vi "New Buffer with data.vi"(7 "#bytes per timestamp":i32, 9 "New Buffer Size (#timestamps)":i32, 10 "Values (buffered, rotated)":u8[](array[numeric]), 11 "Timestamps (buffered, rotated)":u64[](array[numeric])) -> (0 "Full?":bool, 1 "index":i32, 2 "Values (new buffer)":u8[](array[numeric]), 3 "Timestamps (new buffer)":u64[](array[numeric]))   [LabVIEW 2021, in "Ring Buffer Time Series Data.lvlib"]
uses:
  Ring Buffer Time Series Data.lvlib
  Enforce array size multiple timestamps.vi
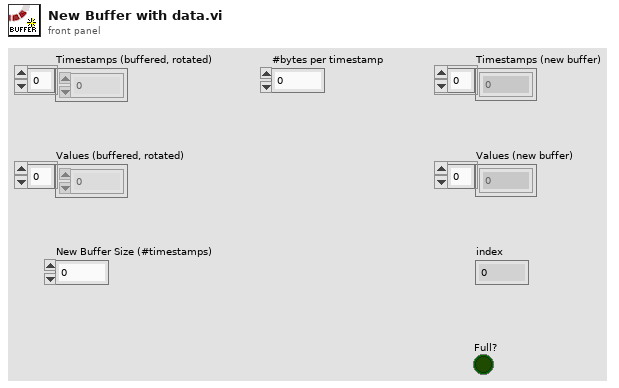
[diagram p1: front panel]
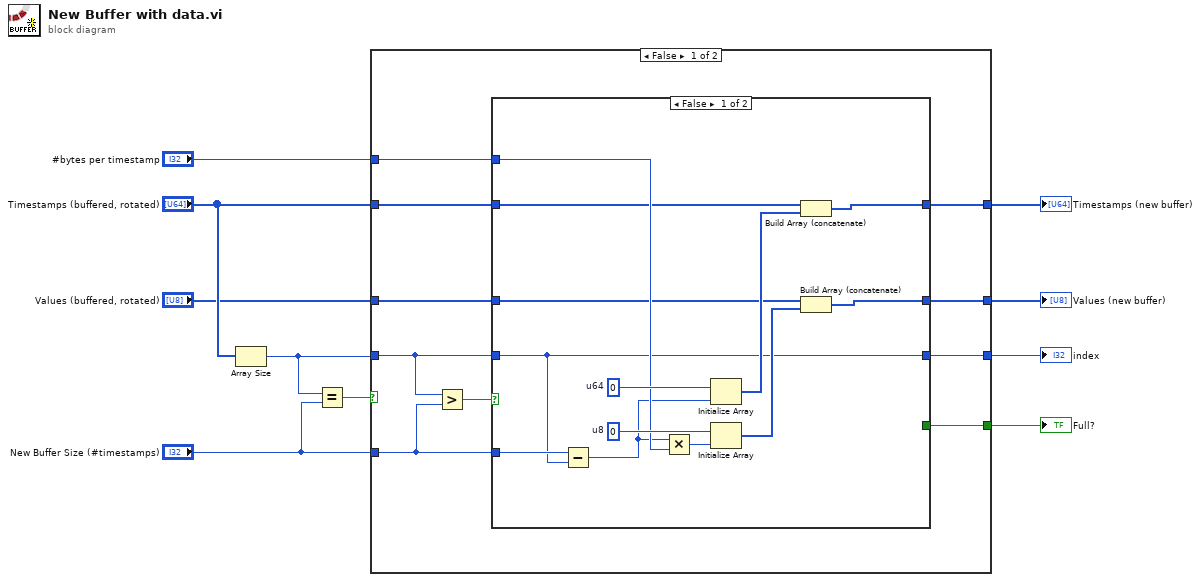
[diagram p0: block diagram]
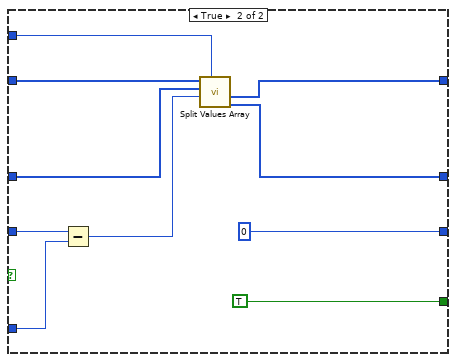
[diagram p2: hidden frame]
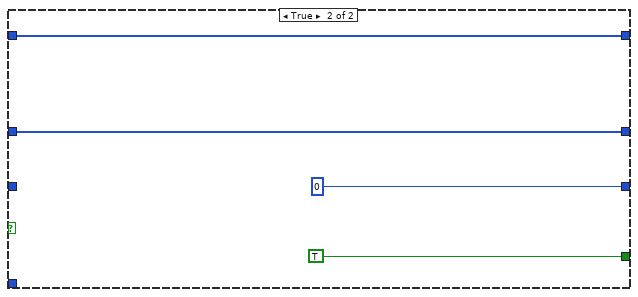
[diagram p3: hidden frame]
diagram:
  n1 = Array Size(array="Timestamps (buffered, rotated)") -> (size(s)=w4:i32)
  n2 = Equal?(x=w4, y="New Buffer Size (#timestamps)") -> (x = y?=w10:bool)
  n3 = case shown="False" w10 {
    tunnel: "Timestamps (buffered, rotated)" -> [w19 w47]
    tunnel: [w18 w47] -> w8
    tunnel: "Values (buffered, rotated)" -> [w16 w46]
    tunnel: [w15 w46] -> w6
    tunnel: [w12 TRUE ("Full?")] -> w5
    tunnel: w4 -> [w11 _]
    tunnel: "New Buffer Size (#timestamps)" -> [w14 _]
    tunnel: "#bytes per timestamp" -> [w17 _]
    tunnel: [w13 0] -> w1
    frame False {
      n4 = Greater?(x=w11, y=w14) -> (0:w20:bool)
      n5 = case shown="False" w20 {
        tunnel: w19 -> [w27 w43]
        tunnel: [w25 w40] -> w18
        tunnel: w17 -> [w29 w42]
        tunnel: w16 -> [w24 w41]
        tunnel: [w22 w39] -> w15
        tunnel: w14 -> [w33 w35]
        tunnel: [w21 0] -> w13
        tunnel: [_ TRUE ("Full?")] -> w12
        tunnel: w11 -> [w21 w36]
        frame False {
          w30 = u64 0  # u64
          w31 = u8 0  # u8
          n6 = Subtract(x=w33, y=w21) -> (x-y=w28:i32)
          n7 = Multiply(x=w28, y=w29) -> (x*y=w32:i32)
          n8 = Initialize Array(w30, w28) -> (w26:u64[])
          n9 = Initialize Array(w31, w32) -> (w23:u8[])
          n10 = Build Array (concatenate)(w27, w26) -> (w25:u64[])
          n11 = Build Array (concatenate)(w24, w23) -> (w22:u8[])
        }
        frame True {
          n12 = Subtract(x=w36, y=w35) -> (x-y=w34:i32)
          n13 = call "Split Values Array.vi"("#bytes per timestamp"=w42, "split index"=w34, "Values"=w41, "Timestamps"=w43) -> ("Values (post-split)"=w39:u8[], "Timestamps (post-split)"=w40:u64[])  [unwired: 4 in, 2 out]
        }
      }
    }
    frame True {
    }
  }
  "Values (new buffer)" <- w6
  "Timestamps (new buffer)" <- w8
  "Full?" <- w5
  "index" <- w1
